vi "Initialize.vi"(5 "Retry Attempts (0)":i32 min=0, 7 "Serial Configuration":T1={"Baud Rate"=9600, "Parity"=0, "Flow Control"=0, "Data Bits"=8, "Stop Bits"=10} {"Stop Bits" items=["1"=10, "1.5"=15, "2"=20]; "Data Bits" items=["8"=8]; "Flow Control" items=["None", "XON/XOFF", "RTS/CTS", "XON/XOFF & RTS/CTS", "DTR/DSR", "XON/XOFF & DTR/DSR"]; "Parity" items=["None"]; "Baud Rate" items=["9600"=9600, "19200"=19200]}, 8 "error in (no error)":errorcluster, 9 "Fast Comms (F)":bool, 11 "VISA resource name":refnum<visa-resource-name>="COM1") -> (0 "error out":errorcluster, 3 "VISA resource name out":refnum<visa-resource-name>)   [LabVIEW 2020, in "driver_chromtech_next_gen.lvlib"]
doc: "Establishes communication with the instrument and optionally performs an instrument identification query and/or an instrument reset. It also places the instrument in a default state needed for other instrument driver operations. Therefore, call this VI before calling other instrument driver VIs for this instrument. Generally, you need to call the <b>Initialize</b> VI only once at the beginning of an application."
uses:
  driver_chromtech_next_gen.lvlib
panel:
  in  "ID Query (F)":bool
  in  "Reset (T)":bool=TRUE
  # "(c) 2021 Iowa State University.  ALL RIGHTS RESERVED."
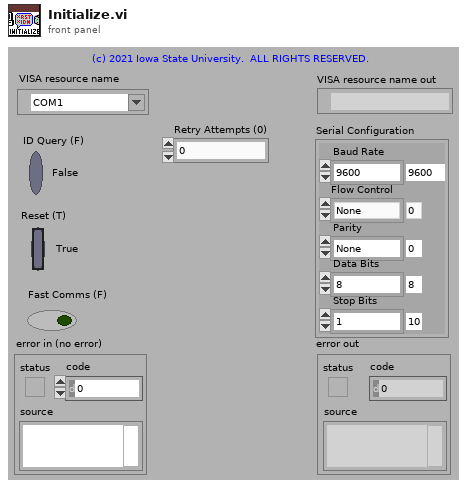
[diagram p1: front panel]
types:
  T1 = cluster{"Baud Rate":u32, "Parity":u16, "Flow Control":u16, "Data Bits":u16, "Stop Bits":u16}
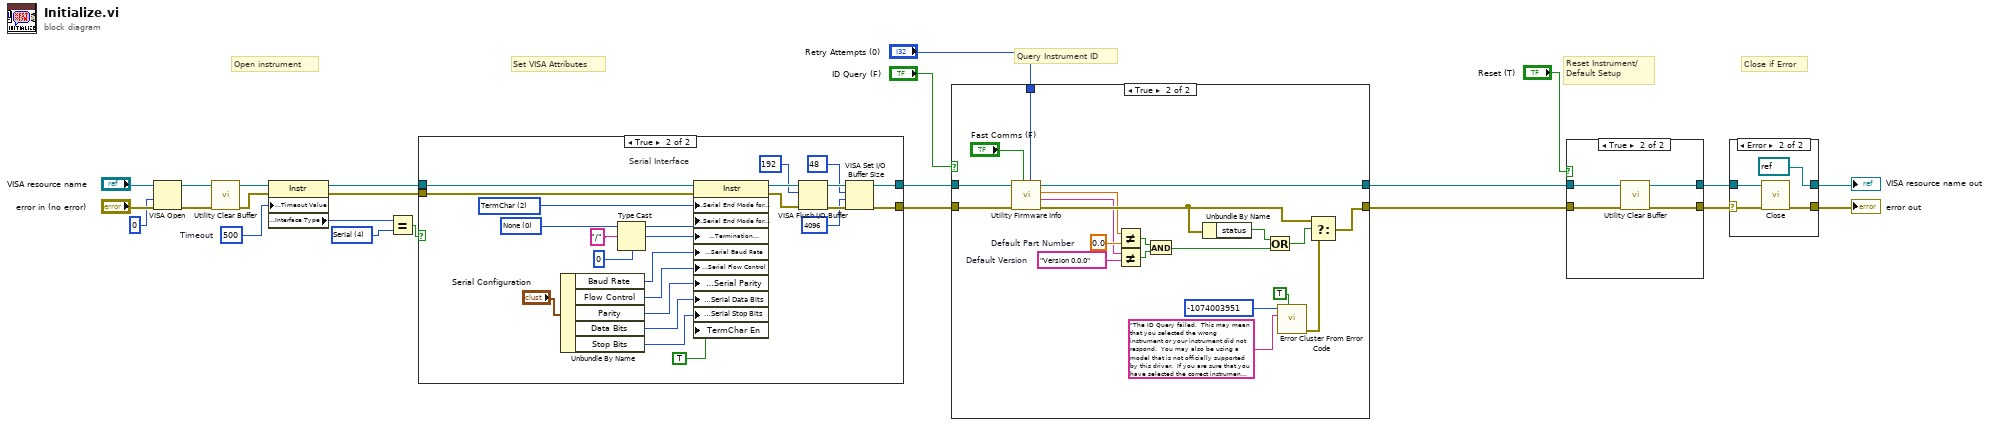
[diagram p0: block diagram]
diagram:
  w16 = u16 4 items=["GPIB"=1, "VXI"=2, "GPIB-VXI"=3, "Serial"=4, "PXI"=5, "TCPIP"=6, "USB"=7] ("Interface Information:Interface Type")
  w20 = u32 500  # Timeout
  # "Query Instrument ID"
  # "Set VISA Attributes"
  # "Close if Error"
  # "Reset Instrument/\nDefault Setup"
  # "Open instrument"
  n1 = VISA Open(access mode=u32 0, error in (no error)="error in (no error)", VISA resource name="VISA resource name") -> (VISA resource name=w14:refnum<visa-resource-name>, error out=w13:errorcluster)  [unwired: 2 in]
  n2 = call "Utility Clear Buffer.vi"("error in (no error)"=w13, "VISA resource name"=w14) -> ("error out"=w11:errorcluster, "VISA resource name out"=w12:refnum<visa-resource-name>)  [unwired: 8 in]
  n3 = property class="Instr"(reference=w12, error in=w11, "General Settings:Timeout Value"=w20) -> (reference out=w19:refnum<visa-resource-name>, error out=w18:errorcluster, "Interface Information:Interface Type"=w21:u16)
  n4 = Equal?(x=w21, y=w16) -> (x = y?=w17:bool)
  n5 = case shown="True" w17 {
    tunnel: [w25 w46] -> w6
    tunnel: [w26 w43] -> w5
    tunnel: w19 -> [w25 w48]
    tunnel: w18 -> [w26 w49]
    frame False {
      # "EDIT: Remove interfaces not supported by your instrument."
      # "GPIB, TCP/IP, and USB Interface"
    }
    frame True {
      w31 = u16 0 items=["None", "LastBit", "TermChar"] ("Serial Settings:Serial End Mode for Reads")
      w38 = u16 2 items=["None", "LastBit", "TermChar"] ("Serial Settings:Serial End Mode for Reads")
      # "Serial Interface"
      n6 = Unbundle By Name("Serial Configuration") -> ("Baud Rate"=w36:u32, "Flow Control"=w33:u16, "Parity"=w35:u16, "Data Bits"=w30:u16, "Stop Bits"=w29:u16)
      n7 = Type Cast(type=u8 0, x="/") -> (*(type *) &x=w37:u8)
      n8 = property class="Instr"(reference=w48, error in=w49, "Serial Settings:Serial End Mode for Reads"=w38, "Serial Settings:Serial End Mode for Writes"=w31, "Message Based Settings:Termination Character"=w37, "Serial Settings:Serial Baud Rate"=w36, "Serial Settings:Serial Flow Control"=w33, "Serial Settings:Serial Parity"=w35, "Serial Settings:Serial Data Bits"=w30, "Serial Settings:Serial Stop Bits"=w29, "TermChar En"=TRUE ("Message Based Settings:Termination Character Enable")) -> (reference out=w42:refnum<visa-resource-name>, error out=w45:errorcluster)
      n9 = VISA Flush I/O Buffer(VISA resource name=w42, mask (16)=u16 192, error in (no error)=w45) -> (VISA resource name out=w47:refnum<visa-resource-name>, error out=w44:errorcluster)
      n10 = VISA Set I/O Buffer Size(VISA resource name=w47, mask (16)=u16 48, size (4096)=u32 4096 ("size (0)"), error in (no error)=w44) -> (VISA resource name out=w46:refnum<visa-resource-name>, error out=w43:errorcluster)
    }
  }
  n11 = case shown="True" "ID Query (F)" {
    tunnel: [w50 w71] -> w4
    tunnel: [w51 w68] -> w3
    tunnel: w6 -> [w51 w69]
    tunnel: w5 -> [w50 w70]
    tunnel: "Retry Attempts (0)" -> [_ w52]
    frame False {
    }
    frame True {
      w58 = "Version 0.0.0"  # Default Version
      w59 = 0.0  # Default Part Number
      n12 = call "Utility Firmware Info.vi"("Retry Attempts (0)"=w52, "Fast Comms (F)"="Fast Comms (F)", "error in"=w70, "VISA resource name"=w69) -> ("error out"=w67:errorcluster, "Firmware Version"=w57:string, "Firmware Part Number"=w60:dbl, "VISA resource name out"=w68:refnum<visa-resource-name>)  [unwired: 4 in]
      n13 = Not Equal?(x=w60, y=w59) -> (x != y?=w55:bool)
      n14 = Not Equal?(x=w57, y=w58) -> (x != y?=w56:bool)
      n15 = And(x=w55, y=w56) -> (x .and. y?=w54:bool)
      n16 = Unbundle By Name(w67) -> ("status"=w62:bool)
      n17 = Or(x=w62, y=w54) -> (x .or. y?=w61:bool)
      n18 = call <vilib>:"Error Cluster From Error Code.vi"("show call chain? (False)"=TRUE, "error message (\"\")"="The ID Query failed.  This may mean that you selected the wrong instrument or your instrument did not respond.  You may also be using a model that is not officially supported by this driver.  If you are sure that you have selected the correct instrument and it is responding, try disabling the ID Query." ("Source (VI Name)"), "error code (0)"=-1074003951 ("Code")) -> ("error out"=w66:errorcluster)  [unwired: 6 in]
      n19 = Select(t=w67, s=w61, f=w66) -> (s? t:f=w71:errorcluster)
    }
  }
  n20 = case shown="True" "Reset (T)" {
    tunnel: w4 -> [w72 w75]
    tunnel: [w72 w74] -> w8
    tunnel: w3 -> [w73 w77]
    tunnel: [w73 w76] -> w9
    frame False {
    }
    frame True {
      n21 = call "Utility Clear Buffer.vi"("error in (no error)"=w75, "VISA resource name"=w77) -> ("error out"=w74:errorcluster, "VISA resource name out"=w76:refnum<visa-resource-name>)  [unwired: 8 in]
    }
  }
  n22 = case shown="Error" w8 {
    selector: w8 -> [w78 w81]
    tunnel: w9 -> [w79 w82]
    tunnel: [w79 refnum<visa-resource-name> refnum ("VISA resource name out")] -> w2
    tunnel: [w78 w83] -> w10
    frame No Error {
    }
    frame Error {
      n23 = call "Close.vi"("error in (no error)"=w81, "VISA resource name"=w82) -> ("error out"=w83:errorcluster)  [unwired: 9 in]
    }
  }
  "VISA resource name out" <- w2
  "error out" <- w10
